vi "Lake Shore 335 Configure Output 2 Advanced Operation.vi"(0 "VISA resource name":refnum<visa-resource-name>) -> ()   [LabVIEW 2015]
doc: "The example demonstrates the proper use of the Configure Heater Output and Configure heater Output 2 Advanced Operation VIs when setting the Warmup Supply and Monitor Output functions. The front panel controls include only the setting that may change when configuring advanced operation."
uses:
  <instrlib>/Lake Shore 335/Lake Shore 335.lvlib
panel:
  in  "Monitor High Value (0.0000)":dbl format="%.4f"
  in  "Monitor Low Value (0.0000)":dbl format="%.4f"
  in  "Monitor Units (1:Kelvin)":u16(ring)=1 items=["Kelvin"=1, "Celsius"=2, "Sensor Units"=3]
  in  "Percentage of Full Scale (0.00 %)":dbl format="%.2f"
  in  "Control (0:Auto Off)":u16(ring) items=["Auto Off", "Continuous"]
  in  "Serial Configuration":T1={"Baud Rate"=57600, "Parity"=1, "Data Bits"=7, "Stop Bits"=10, "Flow Control"=0} {"Flow Control" items=["None", "XON/XOFF", "RTS/CTS", "XON/XOFF & RTS/CTS", "DTR/DSR", "XON/XOFF & DTR/DSR"]; "Stop Bits" items=["1.0"=10, "1.5"=15, "2.0"=20]; "Data Bits" items=["7"=7, "8"=8]; "Parity" items=["None", "Odd", "Even", "Mark", "Space"]; "Baud Rate" items=["300"=300, "600"=600, "1200"=1200, "2400"=2400, "4800"=4800, "9600"=9600, "19200"=19200, "38400"=38400, "57600"=57600]}
  in  "Polarity (0:Unipolar)":u16(ring) items=["Unipolar", "Bipolar"]
  in  "Mode (0:Off)":u16(ring)=4 items=["Off", "Closed Loop PID", "Zone", "Open Loop", "Monitor Out", "Warmup Supply"]
  in  "Power Up Enable (F: Off)":bool
  in  "Input (0:None)":u16(ring) items=["None", "A", "B"]
  # "(c) 2011 Lake Shore Cryotronics Inc.  ALL RIGHTS RESERVED."
  # "Heater Output Settings"
  # "Monitor Output Settings (Mode = Monitor Out, Output Type = Voltage)"
  # "Warmup Supply Settings (Mode = Warmup Supply, Output Type = Voltage)"
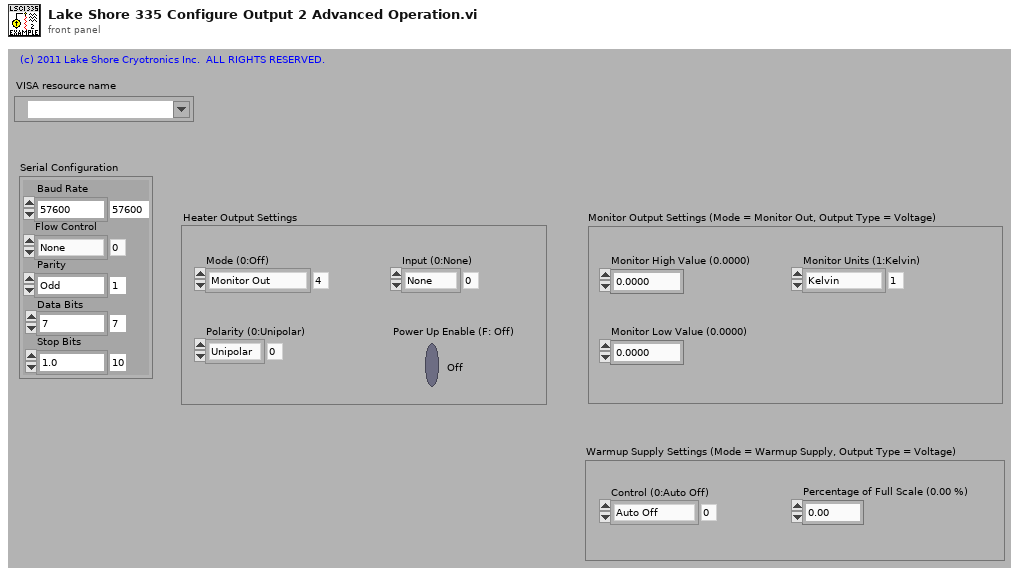
[diagram p1: front panel]
types:
  T1 = cluster{"Baud Rate":u32, "Parity":u16, "Data Bits":u16, "Stop Bits":u16, "Flow Control":u16}
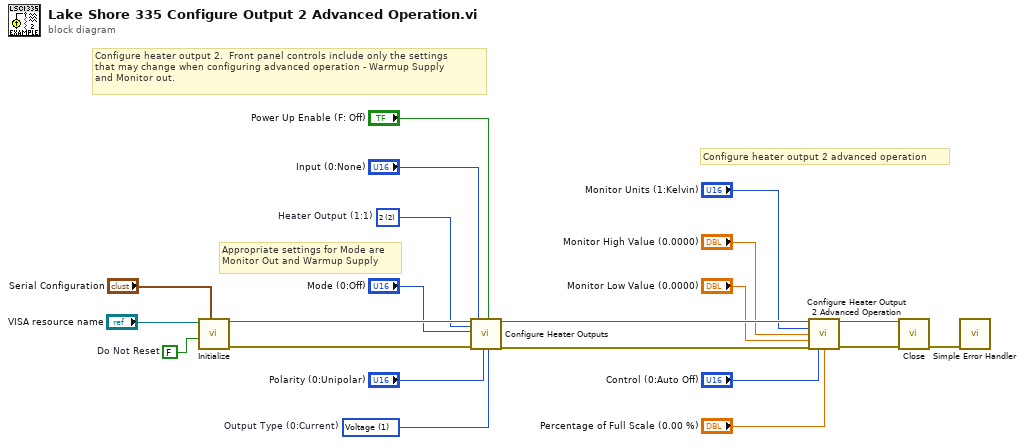
[diagram p0: block diagram]
diagram:
  w1 = u16 1 items=["Current", "Voltage"]  # Output Type (0:Current)
  w2 = u16 2 items=["1"=1, "2"=2]  # Heater Output (1:1)
  w5 = FALSE  # Do Not Reset
  # "Configure heater output 2 advanced operation"
  # "Appropriate settings for Mode are\nMonitor Out and Warmup Supply"
  # "Configure heater output 2.  Front panel controls include only the settings\nthat may change when configuring advanced operation - Warmup Supply\nand Monitor out."
  n1 = call <instrlib>:"Initialize.vi"("Serial Configuration"="Serial Configuration", "Reset (True)"=w5, "VISA resource name"="VISA resource name") -> ("error out"=w19:errorcluster, "VISA resource name out"=w20:refnum<visa-resource-name>)  [unwired: 7 in]
  n2 = call <instrlib>:"Configure Heater Outputs.vi"("VISA resource name"=w20, "Heater Output (1:1)"=w2, "Mode (0:Off)"="Mode (0:Off)", "error in (no error)"=w19, "Input (0:None)"="Input (0:None)", "Polarity (0:Unipolar)"="Polarity (0:Unipolar)", "Power Up Enable (F: Off)"="Power Up Enable (F: Off)", "Output Type (0:Current)"=w1) -> ("VISA resource name out"=w14:refnum<visa-resource-name>, "error out"=w13:errorcluster)  [unwired: 10 in]
  n3 = call <instrlib>:"Configure Heater Output 2 Advanced Operation.vi"("VISA resource name"=w14, "Monitor Units (1:Kelvin)"="Monitor Units (1:Kelvin)", "Monitor High Value (0.0000)"="Monitor High Value (0.0000)", "Monitor Low Value (0.0000)"="Monitor Low Value (0.0000)", "error in (no error)"=w13, "Control (0:Auto Off)"="Control (0:Auto Off)", "Percentage of Full Scale (0.00 %)"="Percentage of Full Scale (0.00 %)") -> ("VISA resource name out"=w12:refnum<visa-resource-name>, "error out"=w11:errorcluster)  [unwired: 7 in]
  n4 = call <instrlib>:"Close.vi"("error in (no error)"=w11, "VISA resource name"=w12) -> ("error out"=w3:errorcluster)  [unwired: 9 in]
  n5 = call <vilib>:"Simple Error Handler.vi"("error in (no error)"=w3) -> ()  [unwired: 4 in, 5 out]
